vi "Comm Interface.vi"(7 "RS-232 Mode (1:Remote)":u16(ring)=1 items=["Local", "Remote", "Locked Remote"], 8 "error in (no error)":errorcluster, 10 "Set/Check (F:Set)":bool, 11 "VISA Resource Name":refnum<visa-resource-name>) -> (0 "error out":errorcluster, 2 "System Interface?":string, 3 "VISA Resource Name Out":refnum<visa-resource-name>)   [LabVIEW 2016, in "Agilent 34970.lvlib"]
doc: "This VI allows you to set or check the instrument's communication interface. You can set the local/remote mode for RS232 communication."
uses:
  Agilent 34970.lvlib
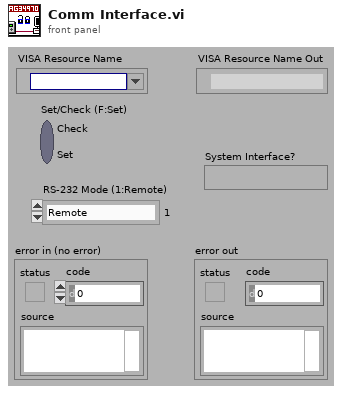
[diagram p1: front panel]
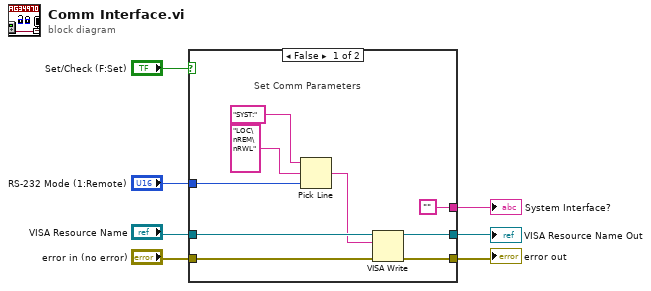
[diagram p0: block diagram]
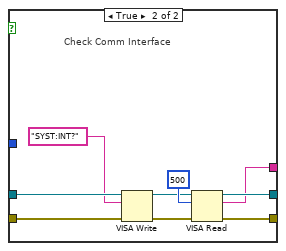
[diagram p2: hidden frame]
diagram:
  n1 = case shown="False" "Set/Check (F:Set)" {
    tunnel: "RS-232 Mode (1:Remote)" -> [w9 _]
    tunnel: "error in (no error)" -> [w16 w21]
    tunnel: [w15 w20] -> w4
    tunnel: [w14 w19] -> w3
    tunnel: "VISA Resource Name" -> [w13 w22]
    tunnel: ["" w18] -> w5
    frame False {
      # "Set Comm Parameters"
      n2 = Pick Line(string ("")="SYST:", multi-line string="LOC\nREM\nRWL", line index=w9) -> (output string=w8:string)
      n3 = VISA Write(VISA resource name=w13, write buffer=w8, error in (no error)=w16) -> (VISA resource name out=w15:refnum<visa-resource-name>, error out=w14:errorcluster)  [unwired: 1 out]
    }
    frame True {
      # "Check Comm Interface"
      n4 = VISA Write(VISA resource name=w22, write buffer="SYST:INT?", error in (no error)=w21) -> (VISA resource name out=w24:refnum<visa-resource-name>, error out=w23:errorcluster)  [unwired: 1 out]
      n5 = VISA Read(VISA resource name=w24, byte count=u32 500 ("byte count (0)"), error in (no error)=w23) -> (VISA resource name out=w20:refnum<visa-resource-name>, read buffer=w18:string, error out=w19:errorcluster)  [unwired: 1 out]
    }
  }
  "System Interface?" <- w5
  "error out" <- w3
  "VISA Resource Name Out" <- w4
